vi "add_EndEffectorCommand.vi"(3 "command":string="CMD_CALIBRATE", 4 "id":u32, 5 "msg in":string) -> (2 "msg out":string)   [LabVIEW 2013]
uses:
  Primitives/subs/u32Scalar.vi
  Primitives/subs/stringScalar.vi
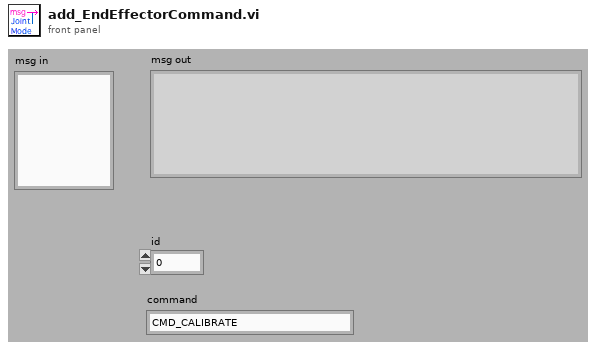
[diagram p1: front panel]
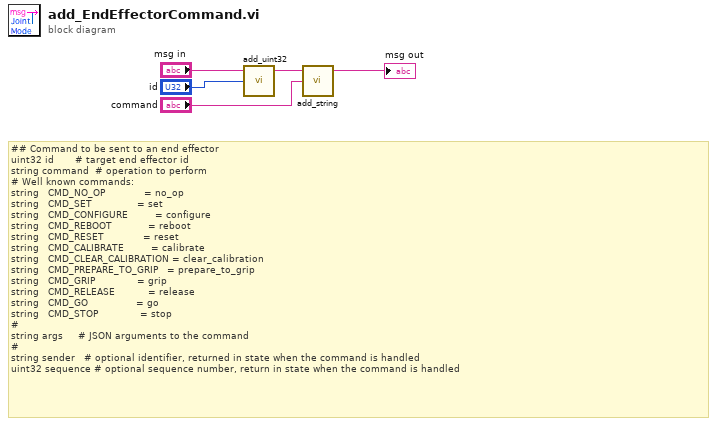
[diagram p0: block diagram]
diagram:
  # "## Command to be sent to an end effector\nuint32 id       # target end effector id\nstring command  # operation to perform\n# Well known commands:\nstring   CMD_NO_OP             = no_op\nstring   CMD_SET               = set\nstring   CMD_CONFIGURE         = configure\nstring   CMD_REBOOT            = reboot\nstring   CMD_RESET             = reset\nstring   CMD_CALIBRATE         = calibrate\nstring   CMD_CLEAR_CALIBRATION = clear_calibration\nstring   CMD_PREPARE_TO_GRIP   = prepare_to_grip\nstring   CMD_GRIP              = grip\nstring   CMD_RELEASE           = release\nstring   CMD_GO                = go\nstring   CMD_STOP              = stop\n#\nstring args     # JSON arguments to the command\n#\nstring sender   # optional identifier, returned in state when the command is handled\nuint32 sequence # optional sequence number, return in state when the command is handled"
  n1 = call-poly "add_uint32.vi"("Numeric"="id", "msg in"="msg in") -> ("msg out"=w5:string)  [unwired: 3 in]
  n2 = call-poly "add_string.vi"("String"="command", "msg in"=w5) -> ("msg out"=→"msg out":string)  [unwired: 3 in]
